vi "Condition VIs.vi"(6 "Msg Output All Terminals":i32[](array[numeric]), 8 "error in":errorcluster, 9 "Msg All Terminals":i32[](array[numeric]), 10 "VI Refs":T1) -> (0 "error out":errorcluster)   [LabVIEW 2025, in "_Msg Rescript.lvlib" / "_Msg Rescript.lvclass"]
uses:
  _Msg Rescript.lvclass
  VI Refs.ctl
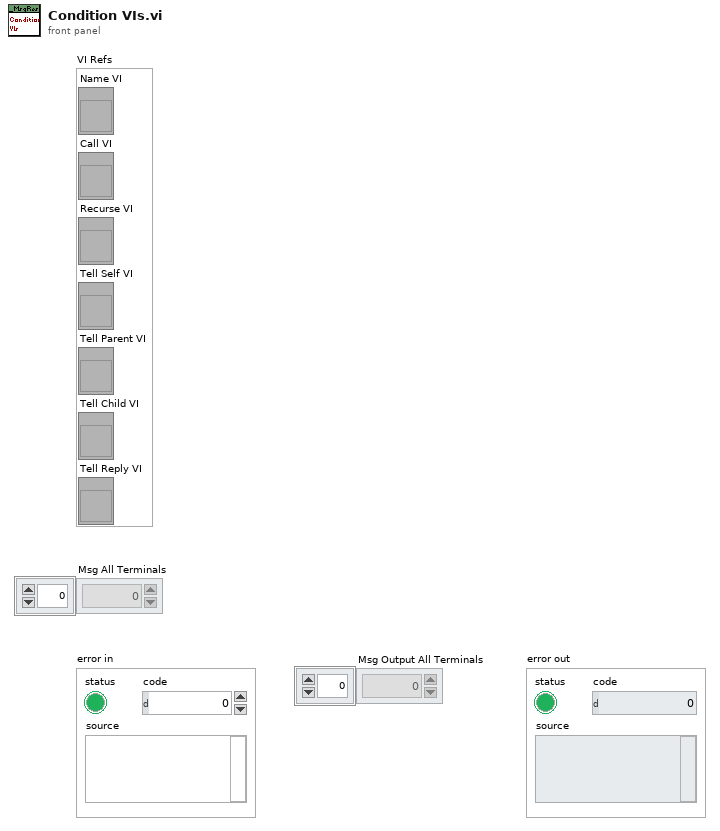
[diagram p1: front panel]
types:
  T1 = typedef "_Msg Rescript.lvlib/_Msg Rescript.lvclass/VI Refs.ctl" = cluster{"Name VI":refnum<vi>, "Call VI":refnum<vi>, "Recurse VI":refnum<vi>, "Tell Self VI":refnum<vi>, "Tell Parent VI":refnum<vi>, "Tell Child VI":refnum<vi>, "Tell Reply VI":refnum<vi>}
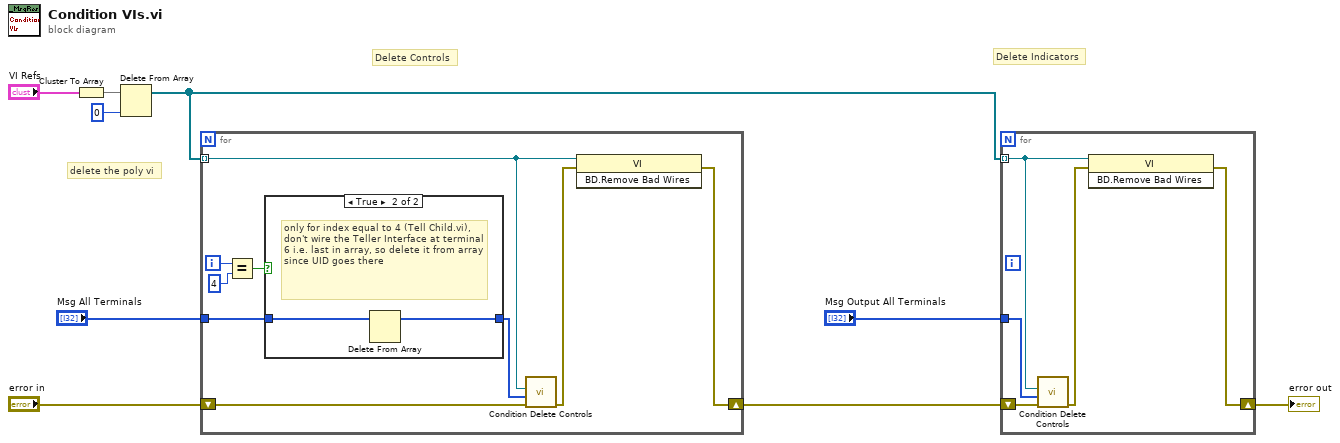
[diagram p0: block diagram]
diagram:
  # "delete the poly vi"
  # "Delete Indicators"
  # "Delete Controls"
  n1 = Cluster To Array(cluster="VI Refs") -> (array=w5:refnum<vi>[])
  n2 = Delete From Array(array=w5, index=0) -> (array with subset deleted=w4:refnum<vi>[])  [unwired: 1 in, 1 out]
  n3 = for {
    tunnel: "Msg All Terminals" -> [w11]
    shift-right: [w16] -> w7
    shift-left: "error in" -> [w18]
    tunnel: w4 -> [w15] mode=indexing
    i -> [w12]
    n4 = Equal?(x=w12, y=4) -> (x = y?=w14:bool)
    n5 = case shown="True" w14 {
      tunnel: w11 -> [w19 w21]
      tunnel: [w19 w20] -> w10
      frame False {
      }
      frame True {
        # "only for index equal to 4 (Tell Child.vi), don't wire the Teller Interface at terminal 6 i.e. last in array, so delete it from array since UID goes there"
        n6 = Delete From Array(array=w21) -> (array with subset deleted=w20:i32[])  [unwired: 2 in, 1 out]
      }
    }
    n7 = call "Condition Delete Controls.vi"("error in"=w18, "Control Terminals"=w10, "VI Ref"=w15) -> ("error out"=w17:errorcluster)  [unwired: 8 in]
    n8 = invoke class="VI" method="BD.Remove Bad Wires"(reference=w15, error in=w17) -> (error out=w16:errorcluster)  [unwired: 1 in, 2 out]
  }
  n9 = for {
    tunnel: "Msg Output All Terminals" -> [w22]
    shift-right: [w24] -> w6
    shift-left: w7 -> [w26]
    tunnel: w4 -> [w23] mode=indexing
    n10 = call "Condition Delete Controls.vi"("error in"=w26, "Control Terminals"=w22, "VI Ref"=w23) -> ("error out"=w25:errorcluster)  [unwired: 8 in]
    n11 = invoke class="VI" method="BD.Remove Bad Wires"(reference=w23, error in=w25) -> (error out=w24:errorcluster)  [unwired: 1 in, 2 out]
  }
  "error out" <- w6
